vi "Debug Exercise (Main).vi"() -> ()   [LabVIEW 2011]
doc: "This VI is an exercise in the LabVIEW Core I course.\n\nThis exercise is used to demonstrate the use of different debugging tools. First, fix the broken run arrow and then use the different debugging tools to see how they work."
panel:
  out "Final Result":dbl format="%.2f"
  out "Random Number":dbl format="%.2f"
  out "Multiply Result":dbl format="%.2f"
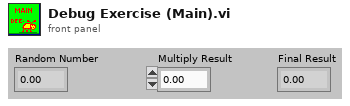
[diagram p1: front panel]
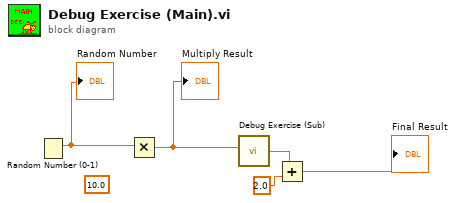
[diagram p0: block diagram]
diagram:
  (unwired) 10.0
  n1 = Random Number (0-1)() -> (number: 0 to 1=w4:dbl)
  "Random Number" <- w4
  n2 = Multiply(x=w4) -> (x*y=w5:dbl)  [unwired: 1 in]
  "Multiply Result" <- w5
  n3 = call "Debug Exercise (Sub).vi"("Number"=w5) -> ("Final Result"=w1:dbl)
  n4 = Add(x=w1, y=2.0) -> (x+y=→"Final Result":dbl)
